vi "getTDMSFilePath.vi"(8 "error in (no error)":errorcluster, 10 "sourceFolder":path, 11 "moveFolder":path) -> (0 "error out":errorcluster, 3 "tdmsFilePath":path)   [LabVIEW 2018]
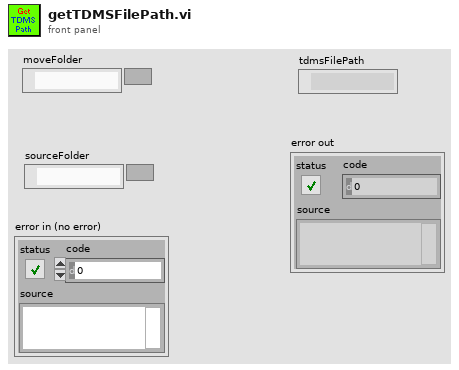
[diagram p1: front panel]
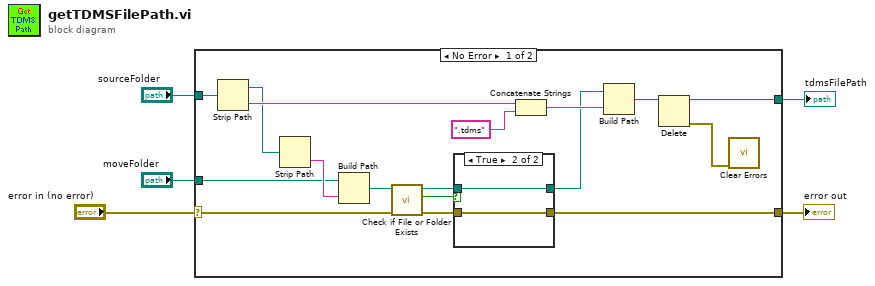
[diagram p0: block diagram]
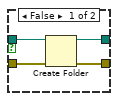
[diagram p2: hidden frame]
diagram:
  n1 = case shown="No Error" "error in (no error)" {
    selector: "error in (no error)" -> [w10 w29]
    tunnel: [w9 w29] -> w4
    tunnel: [w8 _] -> w3
    tunnel: "sourceFolder" -> [w7 _]
    tunnel: "moveFolder" -> [w6 _]
    frame No Error {
      n2 = Strip Path(path=w7) -> (stripped path=w20:path, name=w21:string)
      n3 = Strip Path(path=w20) -> (name=w19:string)  [unwired: 1 out]
      n4 = Build Path(base path=w6, name or relative path=w19) -> (appended path=w17:path)
      n5 = call <vilib>:"Check if File or Folder Exists.vi"("error in (no error)"=w10, "path"=w17) -> ("error out"=w14:errorcluster, "file or folder exists?"=w16:bool, "dup path"=w15:path)  [unwired: 7 in]
      n6 = case shown="True" w16 {
        tunnel: w15 -> [w26 w28]
        tunnel: w14 -> [w25 w27]
        tunnel: [w24 w28] -> w13
        tunnel: [w23 w27] -> w9
        frame False {
          n7 = Create Folder(path (use dialog)=w26, error in=w25) -> (created path=w24:path, error out=w23:errorcluster)  [unwired: 1 in, 1 out]
        }
        frame True {
        }
      }
      n8 = Concatenate Strings(w21, ".tdms" ("x")) -> (w18:string)
      n9 = Build Path(base path=w13, name or relative path=w18) -> (appended path=w12:path)
      n10 = Delete(path (use dialog)=w12) -> (deleted path=w8:path, error out=w11:errorcluster)  [unwired: 4 in, 1 out]
      n11 = call <vilib>:"Clear Errors.vi"("error in (no error)"=w11) -> ()  [unwired: 5 in, 2 out]
    }
    frame Error {
    }
  }
  "error out" <- w4
  "tdmsFilePath" <- w3
